vi "CreateSetupDUTDisplayData.vi"(7 "SMU":T2, 10 "SMU Data":dbl[][](array[numeric]), 11 "DUT Names":string[][](array[string])) -> (3 "DUT Display Data":T1[](array[typedef]) {"Resistance (Ohm)" format="%_4p"; "Current (A)" format="%_4p"; "Voltage (V)" format="%_4p"})   [LabVIEW 2013]
uses:
  driver/Public/Controls/SMU.ctl
  DUTDisplayData.ctl
  driver/Keithley-2602.lvlib
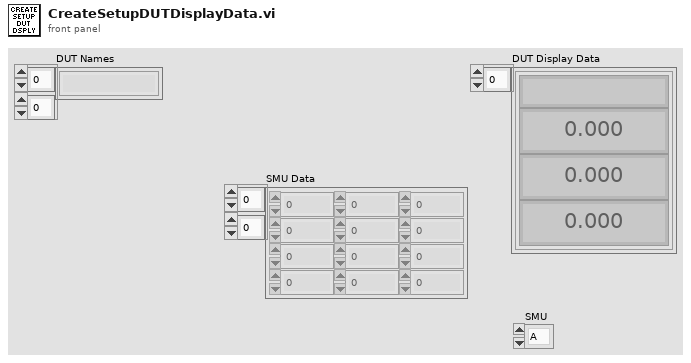
[diagram p1: front panel]
types:
  T1 = typedef "DUTDisplayData.ctl" = cluster{"Name":string, "Voltage (V)":dbl, "Current (A)":dbl, "Resistance (Ohm)":dbl}
  T2 = typedef "Keithley-2602.lvlib/SMU.ctl" = enum16{"A", "B"}
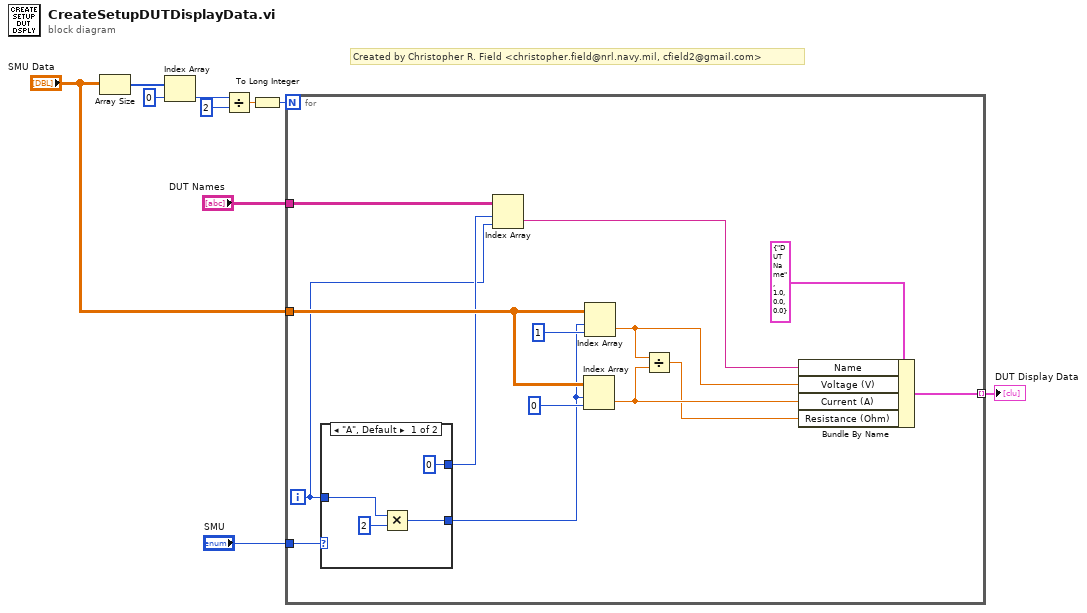
[diagram p0: block diagram]
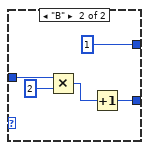
[diagram p2: hidden frame]
diagram:
  # "Created by Christopher R. Field <christopher.field@nrl.navy.mil, cfield2@gmail.com>"
  n1 = Array Size(array="SMU Data") -> (size(s)=w10:i32[])
  n2 = Index Array(array=w10, index=0) -> (element=w8:i32)
  n3 = Divide(x=w8, y=2) -> (x/y=w3:dbl)
  n4 = To Long Integer(number=w3) -> (32bit integer=w4:i32)
  n5 = for {
    N: w4 -> [_]
    tunnel: "SMU Data" -> [w24]
    tunnel: "SMU" -> [w21]
    tunnel: [w16] -> w1 mode=indexing
    tunnel: "DUT Names" -> [w15]
    i -> [w13]
    n6 = case shown="\"A\", Default" w21 {
      tunnel: [w27 w31] -> w20
      tunnel: w13 -> [w26 w33]
      tunnel: [0 1] -> w14
      frame "A", Default {
        n7 = Multiply(x=w26, y=u32 2) -> (x*y=w27:u32)
      }
      frame "B" {
        n8 = Multiply(x=w33, y=u32 2) -> (x*y=w30:u32)
        n9 = Increment(x=w30) -> (x+1=w31:u32)
      }
    }
    n10 = Index Array(array=w15, index (row)=w14, index (col)=w13) -> (element=w12:string)
    n11 = Index Array(array=w24, index (row)=w20, index (col)=0 ("disabled index (col)")) -> (element=w17:dbl)
    n12 = Index Array(array=w24, index (row)=w20, index (col)=1 ("disabled index (col)")) -> (element=w18:dbl)
    n13 = Divide(x=w18, y=w17) -> (x/y=w11:dbl)
    n14 = Bundle By Name(cluster=T1 {"Name"="DUT Name", "Voltage (V)"=1.0, "Current (A)"=0.0, "Resistance (Ohm)"=0.0} ("DUT Display Data"), "Name"=w12, "Voltage (V)"=w18, "Current (A)"=w17, "Resistance (Ohm)"=w11) -> (w16:T1)
  }
  "DUT Display Data" <- w1
